vi "exec.vi"(8 "error in (no error)":errorcluster, 10 "context":refnum<class "Context.lvclass">, 11 "ForceDemand in":refnum<class "ForceDemand.lvclass">) -> (0 "error out":errorcluster, 2 "context 2":refnum<class "Context.lvclass">, 3 "ForceDemand out":refnum<class "ForceDemand.lvclass">)   [LabVIEW 2013, in "ForceDemand.lvclass"]
uses:
  ForceDemand.lvclass
  Context/Context.lvclass
  ForceDemand.lvclass/ForceDemand.ctl
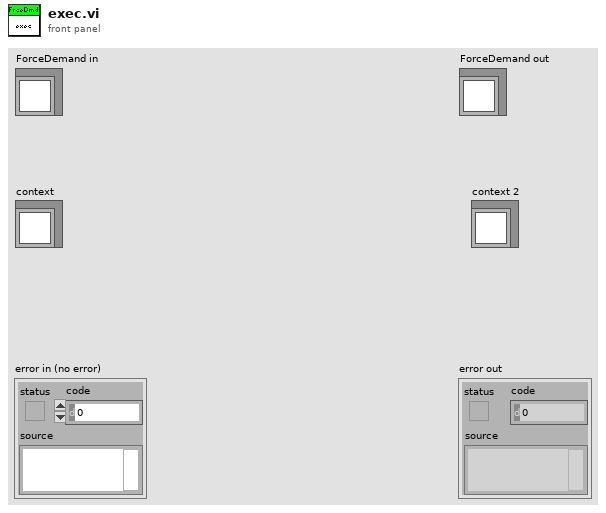
[diagram p1: front panel]
types:
  T1 = typedef "ForceDemand.ctl" = dbl[unit]
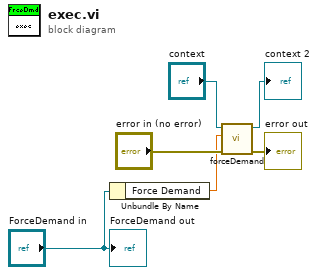
[diagram p0: block diagram]
diagram:
  n1 = Unbundle By Name("ForceDemand in") -> ("Force Demand"=w1:T1)
  n2 = call "forceDemand.vi"("error in (no error)"="error in (no error)", "Force Demand"=w1, "Context in"="context") -> ("error out"=→"error out":errorcluster, "Context out"=→"context 2":refnum<class "Context.lvclass">)  [unwired: 7 in]
  "ForceDemand out" <- "ForceDemand in"
